vi "Lockin_Metrics_Results.vi"() -> ()   [LabVIEW 2013]
uses:
  <vilib>/Analysis/NI_AALPro.lvlib
panel:
  out "Intensity Graph 2":dbl[][](graph)
  out "XY Graph 4":cluster{dbl[], dbl[]}[](graph)
  out "XY Graph 3":cluster{dbl[], "Unwrapped Phase":dbl[]}[](graph)
  out "XY Graph 2":cluster{dbl[], dbl[]}[](graph)
  out "XY Graph":cluster{dbl[], "Unwrapped Phase":dbl[]}[](graph)
  out "Intensity Graph":dbl[][](graph)
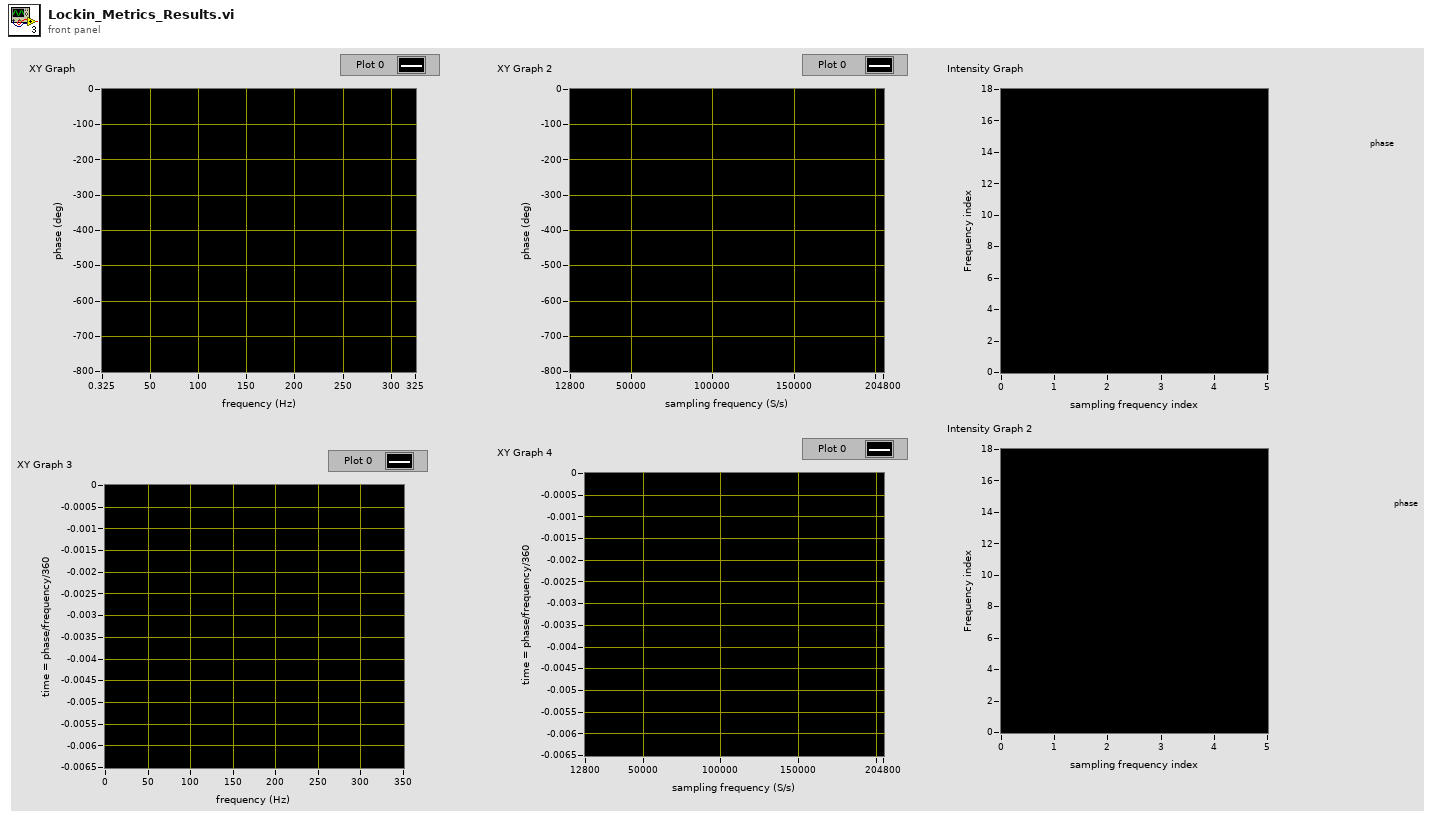
[diagram p1: front panel]
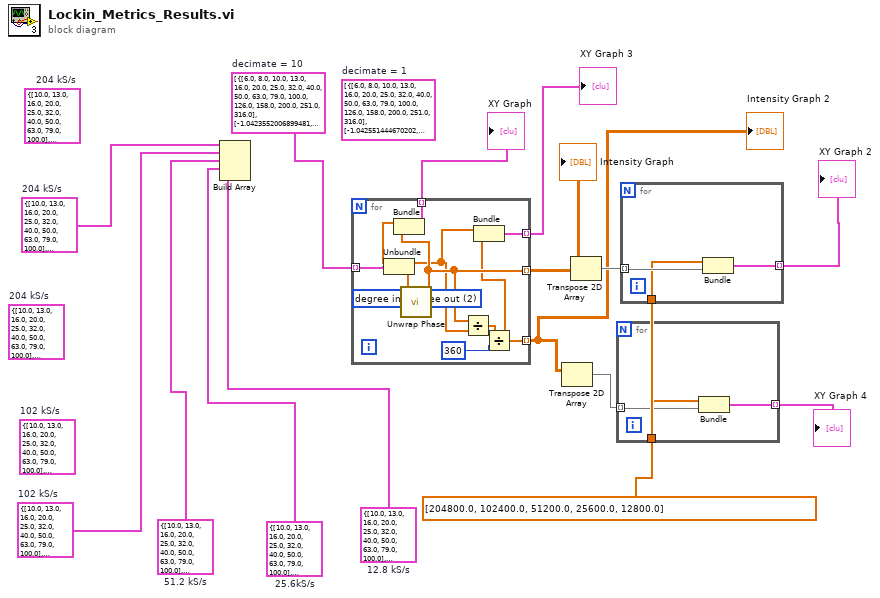
[diagram p0: block diagram]
diagram:
  (unwired) cluster{dbl[], dbl[]}[] [{[6.0, 8.0, 10.0, 13.0, 16.0, 20.0, 25.0, 32.0, 40.0, 50.0, 63.0, 79.0, 100.0, 126.0, 158.0, 200.0, 251.0, 316.0], [-1.042551444670202, -1.390286200596408, -1.7379023644028653, -2.2594885555691557, -2.7806990686890645, -3.475901336106295, -4.344888312497937, -5.561426519993102, -6.9517293607788515, -8.689581511684963, -10.951603505335179, -13.731688221923186, -17.379123396143175, -68.31376629718052, -27.463320797942906, -34.75833613797563, -43.67157184263344, -54.92660931651193]}, {[6.0, 8.0, 10.0, 13.0, 16.0, 20.0, 25.0, 32.0, 40.0, 50.0, 63.0, 79.0, 100.0, 126.0, 158.0, 200.0, 251.0, 316.0], [-2.396228261556458, -3.1950551147975554, -3.994009736815307, -5.192793981289319, -6.390430353298161, -7.98799998895482, -9.984976340244407, -12.780765701529326, -15.975900048886716, -19.96981088918427, -25.168099067334982, -31.557205813729986, -39.93965875872645, -50.367128517504945, -63.11435431224566, -79.87912078342863, -100.48637052469934, -126.22881732878746]}, {[6.0, 8.0, 10.0, 13.0, 16.0, 20.0, 25.0, 32.0, 40.0, 50.0, 63.0, 79.0, 100.0, 126.0, 158.0, 200.0, 251.0, 316.0], [-4.578844507141791, -6.105106674032352, -7.631541737604342, -9.92223318615856, -12.210565534256958, -15.263150450034367, -19.07897293602313, -24.42096540123966, -30.526147882602544, -38.15768263406206, -48.11996197471852, -60.298590435187386, -76.3153655720566, -96.23993645028102, -120.59698178987483, -152.63055352874002, 167.5210016453071, 118.80602671527863]}, {[6.0, 8.0, 10.0, 13.0, 16.0, 20.0, 25.0, 32.0, 40.0, 50.0, 63.0, 79.0, 100.0, 126.0, 158.0, 200.0, 251.0, 316.0], [-7.601510360428238, -10.134012194389173, -12.66764609157601, -16.46995621519307, -20.268335238176093, -25.335462017347343, -31.66925568538951, -40.536584758407265, -50.67079218299738, -63.33837827150104, -79.87496166485602, -100.09019783988313, -126.67665189308948, -159.74979070923206, 159.81960236294395, 106.64668568645395, 38.920525223538384, -40.360678873952274]}, {[6.0, 8.0, 10.0, 13.0, 16.0, 20.0, 25.0, 32.0, 40.0, 50.0, 63.0, 79.0, 100.0, 126.0, 158.0, 200.0, 251.0, 316.0], [-13.308289682876634, -17.74189419027017, -22.177456513967325, -28.848725482018917, -75.64946212867738, -44.35497630174648, -55.44368282798004, -70.96788826070693, -88.70980526878384, -110.88719845818689, -139.8379868730806, -175.22916418357028, 138.22571137866012, 78.9400159278708, 9.541854480959442, -83.54856445090964, 152.26169470097, 10.325367977639084]}]  # decimate = 1
  w6 = cluster{dbl[], dbl[]}[] [{[6.0, 8.0, 10.0, 13.0, 16.0, 20.0, 25.0, 32.0, 40.0, 50.0, 63.0, 79.0, 100.0, 126.0, 158.0, 200.0, 251.0, 316.0], [-1.0423552006899481, -1.3903098827137441, -1.737910087407978, -2.258602969396565, -2.780700875743044, -3.4759131475495986, -4.3427397744037775, -5.561410067975827, -6.951654879976554, -8.663719069464769, -10.951555957699167, -13.711029901411914, -17.246494034944234, -21.778009051453306, -27.24075542599655, -34.5456962508097, -43.31768132301928, -54.27310168510232]}, {[6.0, 8.0, 10.0, 13.0, 16.0, 20.0, 25.0, 32.0, 40.0, 50.0, 63.0, 79.0, 100.0, 126.0, 158.0, 200.0, 251.0, 316.0], [-2.394512524549026, -3.1951138258068474, -3.993858169174312, -5.184745780396297, -6.39037968222766, -7.988004770549838, -9.955466234078624, -12.780709734160709, -15.975883458272529, -19.821353790823995, -25.029673267394205, -31.31604215971608, -39.71735275405901, -50.22855551694198, -62.57103577930017, -79.80881797367354, -100.96616223993937, -143.65396563594373]}, {[6.0, 8.0, 10.0, 13.0, 16.0, 20.0, 25.0, 32.0, 40.0, 50.0, 63.0, 79.0, 100.0, 126.0, 158.0, 200.0, 251.0, 316.0], [-4.575602702700928, -6.105156609854453, -7.631522866632165, -9.881155067562743, -12.210535086383176, -15.263155416275039, -18.935778292399107, -24.420970742609715, -30.526174476673805, -37.93796640098544, -47.979574000445005, -59.711655402974536, -76.21887806944387, -96.51996411683551, -121.26174047622227, -153.59065300624428, 167.97792631895848, 119.38042104141758]}, {[6.0, 8.0, 10.0, 13.0, 16.0, 20.0, 25.0, 32.0, 40.0, 50.0, 63.0, 79.0, 100.0, 126.0, 158.0, 200.0, 251.0, 316.0], [-7.57964181347611, -10.13404641820485, -12.667639885328223, -16.320504761233593, -20.268332509485393, -25.335392935177406, -31.4657202920537, -40.53657512046089, -50.67071796610371, -63.16238008577377, -79.66277443157338, -100.4063846929105, -128.05440476669924, -160.22370990094828, 160.3519081985147, 107.22357024973016, 38.345551664902615, -39.56831452469504]}, {[6.0, 8.0, 10.0, 13.0, 16.0, 20.0, 25.0, 32.0, 40.0, 50.0, 63.0, 79.0, 100.0, 126.0, 158.0, 200.0, 251.0, 316.0], [-13.271355961832105, -17.741847765130448, -22.177434155746315, -28.647526806703006, -35.483952775683804, -44.35492429666974, -55.236018791420086, -70.96784186451556, -88.70976975129923, -111.98836517715236, -140.66909770193755, -175.26530770826307, 141.97077179370692, 78.63856654833467, 9.403374075159826, -84.79451570950859, 152.26167405559266, 10.325496543692617]}]  # decimate = 10
  w3 = dbl[] [204800.0, 102400.0, 51200.0, 25600.0, 12800.0]
  w11 = cluster{dbl[], dbl[]} {[10.0, 13.0, 16.0, 20.0, 25.0, 32.0, 40.0, 50.0, 63.0, 79.0, 100.0], [-22.177347357347077, -28.647453782279452, -35.4839510878745, -44.35490447043462, -55.2359575041674, -70.96782878702648, -88.70970392548786, -111.98829411817022, -140.67082789180142, -175.2674098950837, 141.96810119910498]}  # 12.8 kS/s
  w12 = cluster{dbl[], dbl[]} {[10.0, 13.0, 16.0, 20.0, 25.0, 32.0, 40.0, 50.0, 63.0, 79.0, 100.0], [-12.667649924576203, -16.320531673489988, -20.268349435737342, -25.335395833038287, -31.465718732081122, -40.53659200697804, -50.67070720726345, -63.16238492790555, -79.66275372139346, -100.4063820268297, -128.05438101802272]}  # 25.6kS/s
  w14 = cluster{dbl[], dbl[]} {[10.0, 13.0, 16.0, 20.0, 25.0, 32.0, 40.0, 50.0, 63.0, 79.0, 100.0], [-7.631498730524052, -9.88115868841235, -12.210516068109593, -15.263146135131139, -18.935734053779516, -24.420969723781536, -30.526190503728152, -37.93796340997649, -47.979593217305506, -59.71166312690888, -76.21886205692414]}  # 51.2 kS/s
  w13 = cluster{dbl[], dbl[]} {[10.0, 13.0, 16.0, 20.0, 25.0, 32.0, 40.0, 50.0, 63.0, 79.0, 100.0], [-3.993990975230528, -5.184704759454692, -6.390366377483922, -7.9879887445918305, -9.955498170544626, -63.065489935842436, -15.975898877445644, -19.82136291176446, -25.029664008393457, -31.316055808712957, -39.71736336224215]}  # 102 kS/s
  (unwired) cluster{dbl[], dbl[]} {[10.0, 13.0, 16.0, 20.0, 25.0, 32.0, 40.0, 50.0, 63.0, 79.0, 100.0], [-3.9939506130290696, -5.184682835521029, -6.390403464609181, -7.987955976921996, -9.955466251553414, -63.06546270523142, -15.975883423561923, -19.821369202183313, -25.02967788219486, -31.31601703845939, -39.71733273104706]}  # 102 kS/s
  (unwired) cluster{dbl[], dbl[]} {[10.0, 13.0, 16.0, 20.0, 25.0, 32.0, 40.0, 50.0, 63.0, 79.0, 100.0], [-1.7379422765705368, -2.2585879027094014, -2.7808098919677477, -3.475903511854646, -4.342679691690998, -5.561400216597984, -51.93615751745938, -8.663707641931161, -10.951569814458525, -13.711083801943122, -17.24649772141729]}  # 204 kS/s
  w15 = cluster{dbl[], dbl[]} {[10.0, 13.0, 16.0, 20.0, 25.0, 32.0, 40.0, 50.0, 63.0, 79.0, 100.0], [-1.73788650684728, -2.258566135538428, -2.7807783454477155, -3.47595049415002, -4.342716434021736, -5.561359524614488, -6.951736359782625, -8.663709584170864, -10.951547464512151, -13.711056628140978, -17.246518412398416]}  # 204 kS/s
  (unwired) cluster{dbl[], dbl[]} {[10.0, 13.0, 16.0, 20.0, 25.0, 32.0, 40.0, 50.0, 63.0, 79.0, 100.0], [-1.7377938854520556, -2.258593144393975, -2.780713007230979, -48.47132862596459, -4.342695016279919, -5.561402665168951, -6.9517480333847, -8.663686279486752, -10.951575345656325, -13.710991375008215, -17.246502612239734]}  # 204 kS/s
  n1 = Build Array(w15, w13, w14, w12, w11) -> ()  [unwired: 1 out]
  n2 = for {
    tunnel: w6 -> [w25] mode=indexing
    tunnel: [w21] -> w10 mode=indexing
    tunnel: [w23] -> w7 mode=indexing
    tunnel: [w17] -> w5 mode=indexing
    tunnel: [w16] -> w1 mode=indexing
    w22 = 2 items=["radian in, radian out", "radian in, degree out", "degree in, degree out", "degree in, radian out"] ("phase unit")
    n3 = Unbundle(w25) -> (w18:dbl[], w24:dbl[])
    n4 = call <vilib>:"Unwrap Phase.vi"("phase unit"=w22, "Phase"=w24) -> ("Unwrapped Phase"=w21:dbl[])  [unwired: 8 in, 1 out]
    n5 = Bundle(w18, "Unwrapped Phase"=w21) -> (w23:cluster{dbl[], "Unwrapped Phase":dbl[]})  [unwired: 1 in]
    n6 = Divide(x=w21, y=w18) -> (x/y=w20:dbl[])
    n7 = Divide(x=w20, y=360) -> (x/y=w16:dbl[])
    n8 = Bundle(w18, w16) -> (w17:cluster{dbl[], dbl[]})  [unwired: 1 in]
  }
  "Intensity Graph" <- w10
  "XY Graph" <- w7
  "XY Graph 3" <- w5
  "Intensity Graph 2" <- w1
  n9 = Transpose 2D Array(2D array=w1) -> (transposed array=w4:dbl[][])
  n10 = Transpose 2D Array(2D array=w10) -> (transposed array=w9:dbl[][])
  n11 = for {
    tunnel: w4 -> [w28] mode=indexing
    tunnel: [w27] -> w2 mode=indexing
    tunnel: w3 -> [w26]
    n12 = Bundle(w26, w28) -> (w27:cluster{dbl[], dbl[]})  [unwired: 1 in]
  }
  "XY Graph 4" <- w2
  n13 = for {
    tunnel: w9 -> [w31] mode=indexing
    tunnel: w3 -> [w30]
    tunnel: [w29] -> w8 mode=indexing
    n14 = Bundle(w30, w31) -> (w29:cluster{dbl[], dbl[]})  [unwired: 1 in]
  }
  "XY Graph 2" <- w8
